vi "SwerveChooseBestAngle.vi"(0 "Current Angle (deg) [-180,+180]":dbl format="%#_13g", 1 "Goal Override Angle (deg) [-180,+180]":dbl format="%#_13g", 3 "Goal Override":bool, 5 "Goal Angle (deg) [-180,+180]":dbl format="%#_13g", 11 "Hysteresis (deg)":dbl=10.0 format="%#_13g") -> (4 "Flipped Goal Angle (deg) [-180, +180]":dbl, 6 "Goal Angle (deg) [-180, +180]":dbl, 8 "Flipped Angular Distance (deg)":dbl format="%_4g", 10 "Angular Distance (deg)":dbl format="%_4g", 15 "Flip Drive Motor Direction":bool)   [LabVIEW 2023]
doc: "Based on the Current Angle and the Goal Angle, this VI calulates the signed angular distance. Taking into account the option to invert the direction of the swerve drive motor and always picking the shortest travel distance. The hysteresis prevents undesirable vacillation between angle choices."
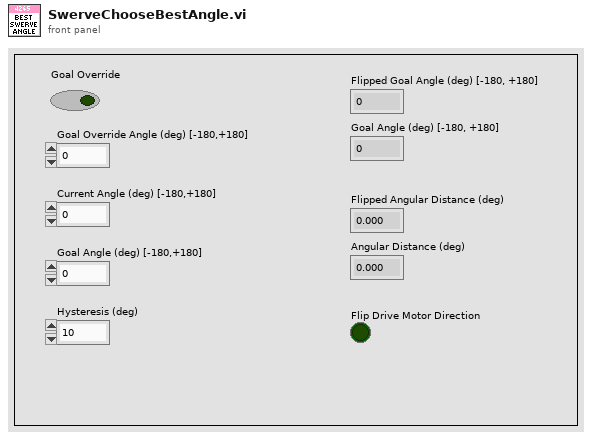
[diagram p1: front panel]
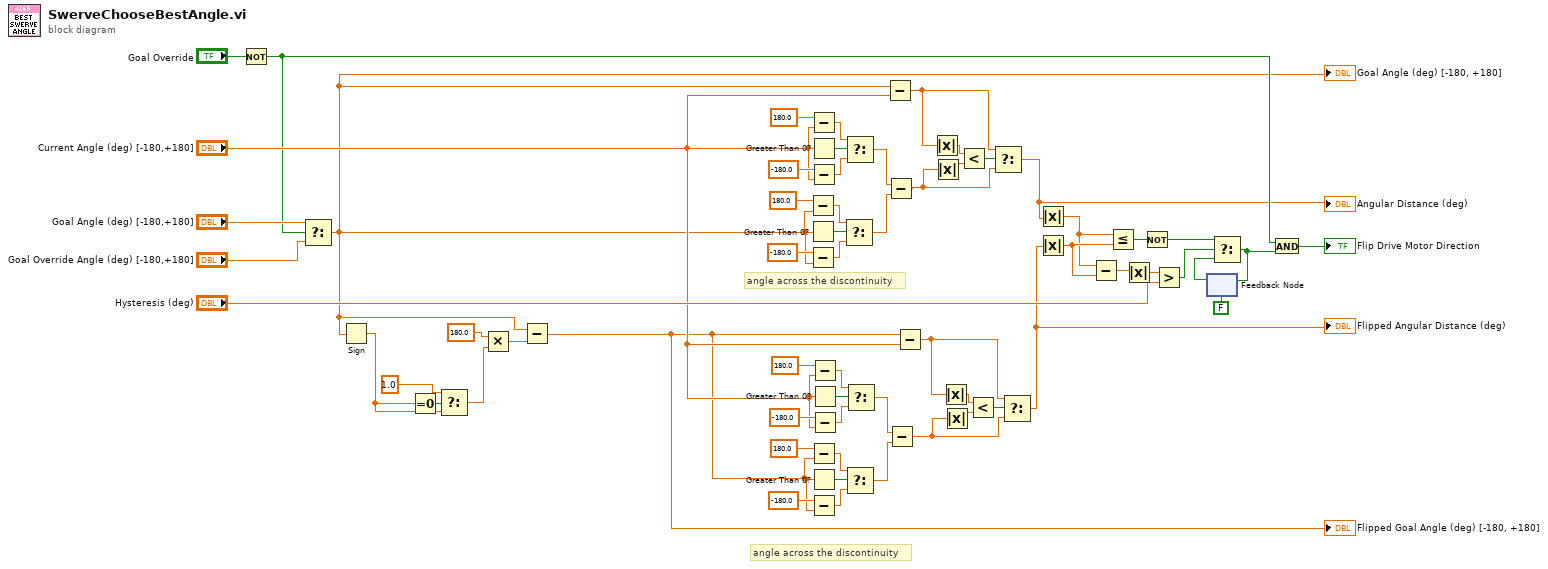
[diagram p0: block diagram]
diagram:
  # "angle across the discontinuity"
  # "angle across the discontinuity"
  n1 = Not(x="Goal Override") -> (.not. x?=w7:bool)
  n2 = Select(t="Goal Angle (deg) [-180,+180]", s=w7, f="Goal Override Angle (deg) [-180,+180]") -> (s? t:f=w3:dbl)
  "Goal Angle (deg) [-180, +180]" <- w3
  n3 = Sign(1:w3) -> (0:w14:dbl)
  n4 = Equal To 0?(x=w14) -> (x = 0?=w15:bool)
  n5 = Select(t=1.0, s=w15, f=w14) -> (s? t:f=w11:dbl)
  n6 = Multiply(x=180.0 ("y"), y=w11) -> (x*y=w61:dbl)
  n7 = Subtract(x=w3, y=w61) -> (x-y=w4:dbl)
  "Flipped Goal Angle (deg) [-180, +180]" <- w4
  n8 = Subtract(x=180.0, y=w3) -> (x-y=w24:dbl)
  n9 = Greater Than 0?(x=w3) -> (x > 0?=w26:bool)
  n10 = Subtract(x=-180.0, y=w3) -> (x-y=w22:dbl)
  n11 = Subtract(x=180.0, y="Current Angle (deg) [-180,+180]") -> (x-y=w29:dbl)
  n12 = Greater Than 0?(x="Current Angle (deg) [-180,+180]") -> (x > 0?=w31:bool)
  n13 = Subtract(x=-180.0, y="Current Angle (deg) [-180,+180]") -> (x-y=w27:dbl)
  n14 = Subtract(x=180.0, y=w4) -> (x-y=w44:dbl)
  n15 = Greater Than 0?(x=w4) -> (x > 0?=w46:bool)
  n16 = Subtract(x=-180.0, y=w4) -> (x-y=w42:dbl)
  n17 = Subtract(x=180.0, y="Current Angle (deg) [-180,+180]") -> (x-y=w50:dbl)
  n18 = Greater Than 0?(x="Current Angle (deg) [-180,+180]") -> (x > 0?=w52:bool)
  n19 = Subtract(x=-180.0, y="Current Angle (deg) [-180,+180]") -> (x-y=w48:dbl)
  n20 = Select(t=w24, s=w26, f=w22) -> (s? t:f=w20:dbl)
  n21 = Select(t=w29, s=w31, f=w27) -> (s? t:f=w21:dbl)
  n22 = Select(t=w44, s=w46, f=w42) -> (s? t:f=w40:dbl)
  n23 = Select(t=w50, s=w52, f=w48) -> (s? t:f=w41:dbl)
  n24 = Subtract(x=w3, y="Current Angle (deg) [-180,+180]") -> (x-y=w32:dbl)
  n25 = Subtract(x=w21, y=w20) -> (x-y=w18:dbl)
  n26 = Subtract(x=w41, y=w40) -> (x-y=w39:dbl)
  n27 = Subtract(x=w4, y="Current Angle (deg) [-180,+180]") -> (x-y=w36:dbl)
  n28 = Absolute Value(x=w32) -> (abs(x)=w33:dbl)
  n29 = Absolute Value(x=w18) -> (abs(x)=w34:dbl)
  n30 = Absolute Value(x=w36) -> (abs(x)=w37:dbl)
  n31 = Absolute Value(x=w39) -> (abs(x)=w38:dbl)
  n32 = Less?(x=w33, y=w34) -> (x < y?=w35:bool)
  n33 = Less?(x=w37, y=w38) -> (x < y?=w47:bool)
  n34 = Select(t=w32, s=w35, f=w18) -> (s? t:f=w1:dbl)
  "Angular Distance (deg)" <- w1
  n35 = Select(t=w36, s=w47, f=w39) -> (s? t:f=w2:dbl)
  "Flipped Angular Distance (deg)" <- w2
  n36 = Absolute Value(x=w1) -> (abs(x)=w53:dbl)
  n37 = Absolute Value(x=w2) -> (abs(x)=w54:dbl)
  n38 = Subtract(x=w53, y=w54) -> (x-y=w58:dbl)
  n39 = Less Or Equal?(x=w53, y=w54) -> (x <= y?=w17:bool)
  n40 = Absolute Value(x=w58) -> (abs(x)=w57:dbl)
  n41 = Not(x=w17) -> (.not. x?=w16:bool)
  n42 = Greater?(x=w57, y="Hysteresis (deg)") -> (0:w55:bool)
  n43 = feedback #1(FALSE) -> (w60:bool)
  n44 = Select(t=w16, s=w55, f=w60) -> (s? t:f=w10:bool)
  n45 = feedback-in #1(w10) -> ()
  n46 = And(x=w7, y=w10) -> (x .and. y?=→"Flip Drive Motor Direction":bool)
